vi "Get_Folders_Client.vi"(0 "Relative Path":path) -> (1 "Folder Names":string[](array[string]), 2 "error out":errorcluster)   [LabVIEW 2011]
uses:
  Anemometry/Anemometry Sub Vis/Globals/Preference_global.vi
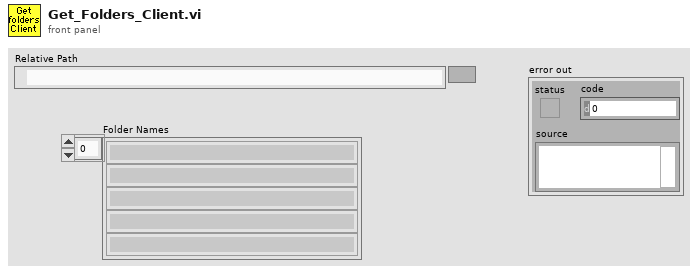
[diagram p1: front panel]
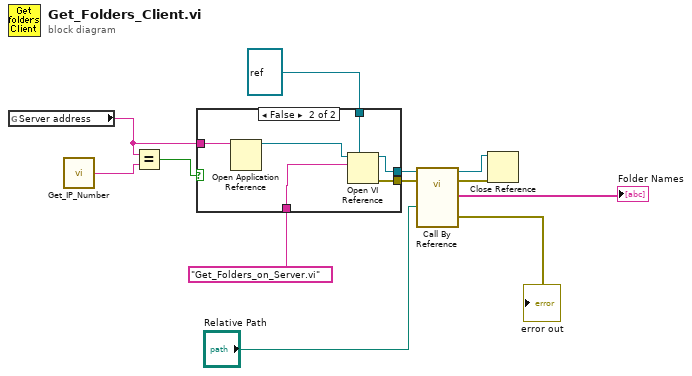
[diagram p0: block diagram]
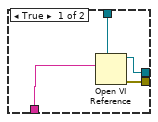
[diagram p2: hidden frame]
diagram:
  n1 = global read "Preference_global.vi" "Server address"() -> (w4:string)
  n2 = call "Get_IP_Number.vi"() -> ("IP Number"=w6:string)
  n3 = Equal?(x=w4, y=w6) -> (x = y?=w5:bool)
  n4 = case shown="False" w5 {
    tunnel: [w16 w22] -> w7
    tunnel: [w15 w21] -> w8
    tunnel: "Get_Folders_on_Server.vi" -> [w14 w20]
    tunnel: refnum<vi> refnum ("Scout Server") -> [w13 w19]
    tunnel: w4 -> [_ w18]
    frame True {
      n5 = Open VI Reference(type specifier VI Refnum (for type only)=w13, vi path=w14) -> (vi reference=w16:refnum<vi>, error out=w15:errorcluster)  [unwired: 2 in, 2 out]
    }
    frame False {
      n6 = Open Application Reference(11:w18) -> (3:w17:refnum<vi>)  [unwired: 2 in, 2 out]
      n7 = Open VI Reference(type specifier VI Refnum (for type only)=w19, application reference (local)=w17, vi path=w20) -> (vi reference=w22:refnum<vi>, error out=w21:errorcluster)  [unwired: 1 in, 2 out]
    }
  }
  n8 = call-by-ref "?"(reference=w7, error in=w8, "Relative Path"="Relative Path") -> (reference out=w9:refnum<vi>, error out=w12:errorcluster, "Folder Names"=→"Folder Names":string[], "error out"=→"error out":errorcluster)  [unwired: 1 in]
  n9 = Close Reference(reference=w9, error in (no error)=w12) -> ()  [unwired: 1 out]
